vi "picoscopeIndividualChannelSettings.vi"(11 "PicoscopeV2 in":refnum<class "PicoscopeV2.lvclass">) -> (3 "PicoscopeV2 out":refnum<class "PicoscopeV2.lvclass">)   [LabVIEW 2020, in "PicoscopeV2.lvclass"]
uses:
  PicoscopeV2.lvclass
  PicoscopeV2.lvclass/PicoscopeV2.ctl
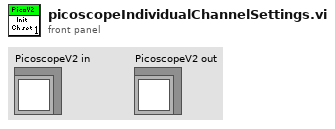
[diagram p1: front panel]
types:
  T1 = typedef "OnOffTypeDef.ctl" = enum16{"off", "on"}
  T2 = typedef "VoltageRange.ctl" = enum16{"10 mV", "20 mV", "50 mV", "100 mV", "200 mV", "500 mV", "1 V", "2 V", "5 V", "10 V", "20 V"}
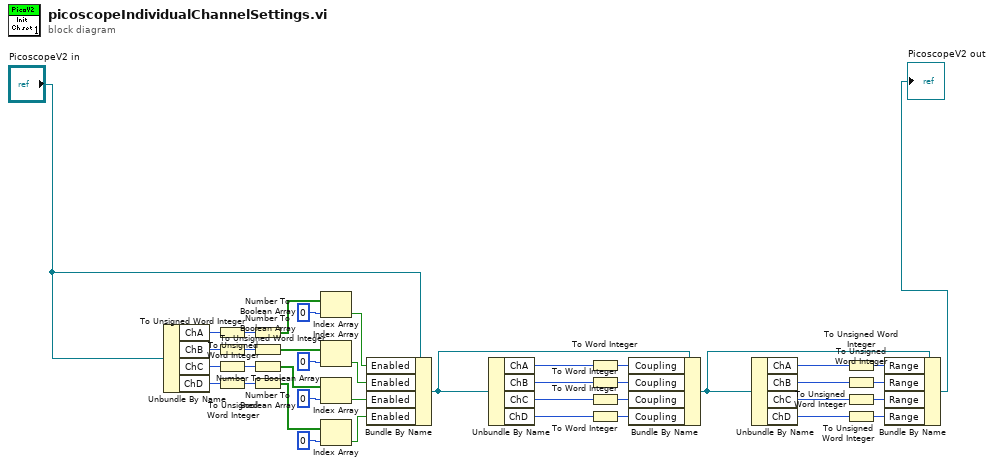
[diagram p0: block diagram]
diagram:
  n1 = Unbundle By Name("PicoscopeV2 in") -> ("ChA"=w39:T1, "ChB"=w35:T1, "ChC"=w34:T1, "ChD"=w33:T1)
  n2 = To Unsigned Word Integer(number=w39) -> (unsigned 16bit integer=w40:u16)
  n3 = To Unsigned Word Integer(number=w35) -> (unsigned 16bit integer=w38:u16)
  n4 = To Unsigned Word Integer(number=w34) -> (unsigned 16bit integer=w37:u16)
  n5 = To Unsigned Word Integer(number=w33) -> (unsigned 16bit integer=w36:u16)
  n6 = Number To Boolean Array(number=w40) -> (Boolean array=w31:bool[])
  n7 = Number To Boolean Array(number=w38) -> (Boolean array=w28:bool[])
  n8 = Number To Boolean Array(number=w37) -> (Boolean array=w26:bool[])
  n9 = Number To Boolean Array(number=w36) -> (Boolean array=w24:bool[])
  n10 = Index Array(array=w31, index=0) -> (element=w30:bool)
  n11 = Index Array(array=w28, index=0) -> (element=w23:bool)
  n12 = Index Array(array=w26, index=0) -> (element=w22:bool)
  n13 = Index Array(array=w24, index=0) -> (element=w21:bool)
  n14 = Bundle By Name(cluster="PicoscopeV2 in", "Enabled"=w30, "Enabled"=w23, "Enabled"=w22, "Enabled"=w21) -> (w11:refnum<class "PicoscopeV2.lvclass">)
  n15 = Unbundle By Name(w11) -> ("ChA"=w20:enum16{"AC", "DC"}, "ChB"=w18:enum16{"AC", "DC"}, "ChC"=w17:enum16{"AC", "DC"}, "ChD"=w16:enum16{"AC", "DC"})
  n16 = To Word Integer(number=w20) -> (16bit integer=w19:i16)
  n17 = To Word Integer(number=w18) -> (16bit integer=w15:i16)
  n18 = To Word Integer(number=w17) -> (16bit integer=w14:i16)
  n19 = To Word Integer(number=w16) -> (16bit integer=w13:i16)
  n20 = Bundle By Name(cluster=w11, "Coupling"=w19, "Coupling"=w15, "Coupling"=w14, "Coupling"=w13) -> (w2:refnum<class "PicoscopeV2.lvclass">)
  n21 = Unbundle By Name(w2) -> ("ChA"=w10:T2, "ChB"=w9:T2, "ChC"=w8:T2, "ChD"=w7:T2)
  n22 = To Unsigned Word Integer(number=w10) -> (unsigned 16bit integer=w6:u16)
  n23 = To Unsigned Word Integer(number=w9) -> (unsigned 16bit integer=w5:u16)
  n24 = To Unsigned Word Integer(number=w8) -> (unsigned 16bit integer=w4:u16)
  n25 = To Unsigned Word Integer(number=w7) -> (unsigned 16bit integer=w3:u16)
  n26 = Bundle By Name(cluster=w2, "Range"=w6, "Range"=w5, "Range"=w4, "Range"=w3) -> (→"PicoscopeV2 out":refnum<class "PicoscopeV2.lvclass">)
